vi "find_element(array).vi"(8 "error in (no error)":errorcluster, 10 "name":string, 11 "data store (in)":cluster{"name":string, "address":string}[](array[cluster])) -> (0 "error out":errorcluster, 1 "element":cluster{"name":string, "address":string}, 2 "element found ?":bool, 3 "data store (out)":cluster{"name":string, "address":string}[](array[cluster]))   [LabVIEW 2016]
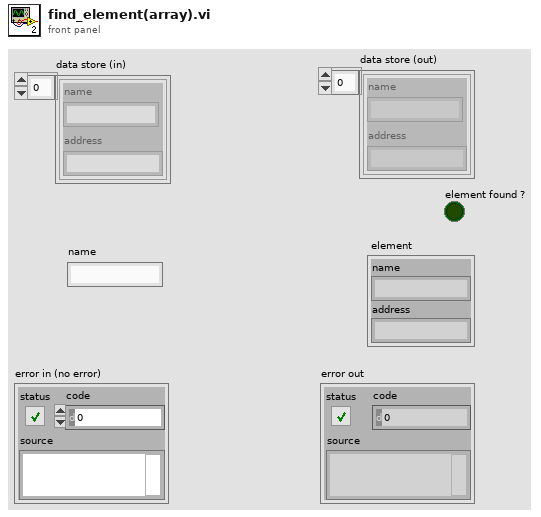
[diagram p1: front panel]
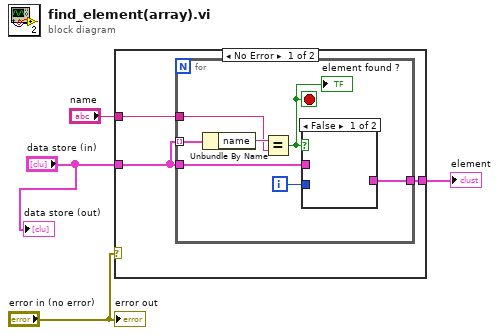
[diagram p0: block diagram]
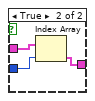
[diagram p2: hidden frame]
diagram:
  n1 = case shown="No Error" "error in (no error)" {
    tunnel: "data store (in)" -> [w6 _]
    tunnel: "name" -> [w7 _]
    tunnel: [w5 _] -> w2
    frame No Error {
      n2 = for {
        tunnel: w6 -> [w14] mode=indexing
        tunnel: w7 -> [w12]
        tunnel: w6 -> [w10]
        tunnel: [w8] -> w5
        i -> [w11]
        stop <- w9 stop-if-true
        n3 = Unbundle By Name(w14) -> ("name"=w13:string)
        n4 = Equal?(x=w13, y=w12) -> (x = y?=w9:bool)
        "element found ?" <- w9
        n5 = case shown="False" w9 {
          tunnel: w11 -> [_ w15]
          tunnel: w10 -> [_ w17]
          tunnel: [_ w16] -> w8
          frame False {
          }
          frame True {
            n6 = Index Array(array=w17, index=w15) -> (element=w16:cluster{"name":string, "address":string})
          }
        }
      }
    }
    frame Error {
    }
  }
  "element" <- w2
  "error out" <- "error in (no error)"
  "data store (out)" <- "data store (in)"
